vi "READ accelerometer.vi"(10 "refnum name":string, 11 "AccelerometerDevRef":T1={"DevStatus"={"status"=FALSE, "code"=0, "source"=""}, "Scaling"={"Gain (VoltsPerG)"=0.0, "Center Voltage"=0.0}, "Analog Channels"={"X-Axis"=enum."AI 0", "Y-Axis"=enum."AI 0", "Z-Axis"=enum."AI 0"}, "I2C Bus"=enum."I2C On-Board", "SPI Bus"=enum."SPI On-Board, CS0", "Accel Range"=0, "ADXL Axes"={"X-Axis"=FALSE, "Y-Axis"=FALSE, "Z-Axis"=FALSE}, "Handle"=0, "Device Address"=0, "Accel Type"=enum."Internal"} {"Device Address" format="%.0x"; "Accel Range" items=["+/- 2 g", "+/- 4 g", "+/- 8 g", "+/- 16 g"]}) -> ()   [LabVIEW 2020]
uses:
  <vilib>/Rock Robotics/WPI/Accelerometer/WPI_AccelerometerDevRef.ctl
  <vilib>/Rock Robotics/WPI/Accelerometer/WPI_AccelerometerScaling.ctl
  <vilib>/Rock Robotics/WPI/Accelerometer/WPI_AccelerometerAnalogChannels.ctl
  <vilib>/Rock Robotics/SystemInterfaces/AI/FPGA_AIChannel.ctl
  <vilib>/Rock Robotics/SystemInterfaces/i2clib/i2c_bus.ctl
  <vilib>/Rock Robotics/SystemInterfaces/spilib/spi_bus.ctl
  <vilib>/Rock Robotics/WPI/Accelerometer/ADXL345 Range.ctl
  <vilib>/Rock Robotics/WPI/Accelerometer/WPI_AccelerometerADXL345 Axes.ctl
  <vilib>/Rock Robotics/Network Tables/NT Write Numeric Array.vi
  <vilib>/Rock Robotics/Network Tables/NT Read Numeric Array.vi
panel:
  # "ADXL"
  # "Analog"
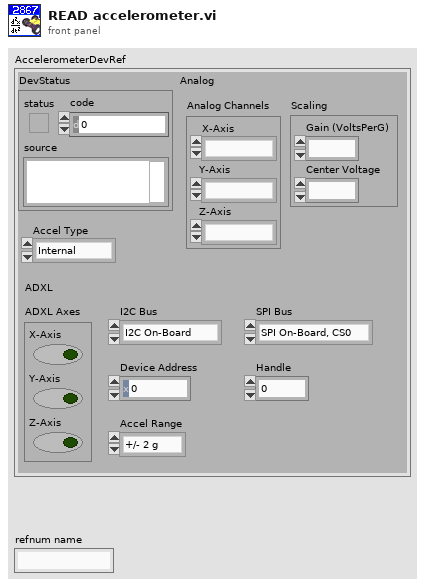
[diagram p1: front panel]
types:
  T1 = typedef "WPI_AccelerometerDevRef.ctl" = cluster{"DevStatus":errorcluster, "Scaling":T2, "Analog Channels":T3, "I2C Bus":T5, "SPI Bus":T6, "Accel Range":T7, "ADXL Axes":T8, "Handle":i32, "Device Address":u8, "Accel Type":enum16{"Analog", "ADXL345 I2C", "ADXL345 SPI", "Internal", "ADXL362 SPI"}}
  T2 = typedef "WPI_AccelerometerScaling.ctl" = cluster{"Gain (VoltsPerG)":dbl, "Center Voltage":dbl}
  T3 = typedef "WPI_AccelerometerAnalogChannels.ctl" = cluster{"X-Axis":T4, "Y-Axis":T4, "Z-Axis":T4}
  T4 = typedef "FPGA_AIChannel.ctl" = enum8{"AI 0", "AI 1", "AI 2", "AI 3", "AI MXP 0", "AI MXP 1", "AI MXP 2", "AI MXP 3", "Invalid"}
  T5 = typedef "i2c_bus.ctl" = enum16{"I2C On-Board", "I2C MXP", "Invalid"}
  T6 = typedef "spi_bus.ctl" = enum16{"SPI On-Board, CS0", "SPI On-Board, CS1", "SPI On-Board, CS2", "SPI On-Board, CS3", "SPI MXP", "Invalid"}
  T7 = typedef "ADXL345 Range.ctl" = u8
  T8 = typedef "WPI_AccelerometerADXL345 Axes.ctl" = cluster{"X-Axis":bool, "Y-Axis":bool, "Z-Axis":bool}
  T9 = cluster{"X-Axis":dbl, "Y-Axis":dbl, "Z-Axis":dbl}
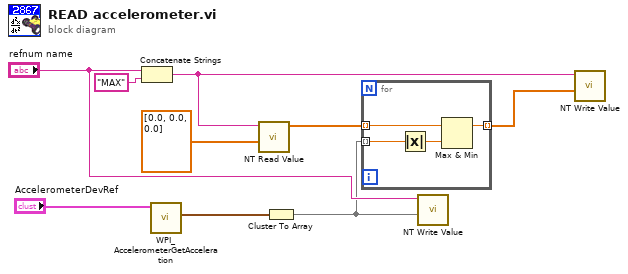
[diagram p0: block diagram]
diagram:
  n1 = Concatenate Strings("refnum name", "MAX" ("string")) -> (w3:string)
  n2 = call <vilib>:"WPI_AccelerometerGetAcceleration.vi"("AccelerometerDevRef"="AccelerometerDevRef") -> ("Accelerations"=w9:T9)  [unwired: 8 in, 2 out]
  n3 = call-poly <vilib>:"NT Read Value.vi"("Default Value"=dbl[] [0.0, 0.0, 0.0] ("array"), "Name"=w3) -> ("Numeric Array"=w5:dbl[])  [unwired: 8 in, 1 out]
  n4 = Cluster To Array(cluster=w9) -> (array=w4:dbl[])
  n5 = for {
    tunnel: w5 -> [w11] mode=indexing
    tunnel: w4 -> [w13] mode=indexing
    tunnel: [w12] -> w2 mode=indexing
    n6 = Absolute Value(x=w13) -> (abs(x)=w10:dbl)
    n7 = Max & Min(x=w11, y=w10) -> (max(x,y)=w12:dbl)  [unwired: 1 out]
  }
  n8 = call-poly <vilib>:"NT Write Value.vi"("Numeric Array"=w4, "Name"="refnum name") -> ()  [unwired: 9 in, 1 out]
  n9 = call-poly <vilib>:"NT Write Value.vi"("Numeric Array"=w2, "Name"=w3) -> ()  [unwired: 9 in, 1 out]
